vi "Acquire.vi"(8 "error in (no error)":errorcluster, 11 "DAQmxAI in":refnum<class "DAQmxAI.lvclass">) -> (0 "error out":errorcluster, 3 "DAQmxAI out":refnum<class "DAQmxAI.lvclass">)   [LabVIEW 2020, in "VolatusDAQ.lvlib" / "DAQmxAI.lvclass"]
uses:
  DAQmxAI.lvclass
  DAQmxAI.lvclass/DAQmxAI.ctl
  <vilib>/DAQmx/read.llb/DAQmx Read (Analog 1D Wfm NChan NSamp).vi
  <vilib>/DAQmx/miscellaneous.llb/DAQmx Fill In Error Info.vi
  VolatusData/VolatusData.lvlib
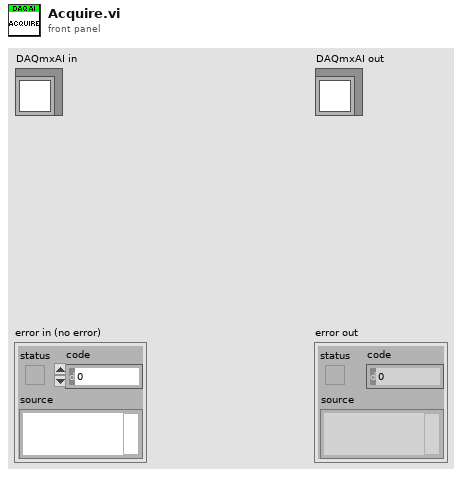
[diagram p1: front panel]
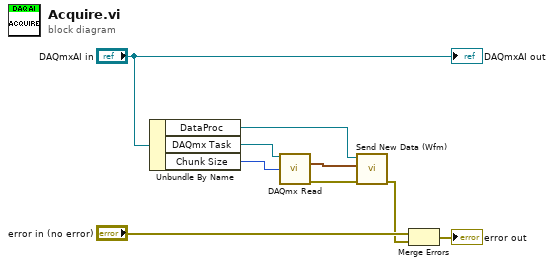
[diagram p0: block diagram]
diagram:
  n1 = Unbundle By Name("DAQmxAI in") -> ("DataProc"=w6:refnum<class "MessageQ.lvclass">, "DAQmx Task"=w8:refnum<k21>, "Chunk Size"=w7:i32)
  n2 = call-poly <vilib>:"DAQmx Read.vi"("task/channels in"=w8, "number of samples per channel"=w7) -> ("data"=w5:waveform(dbl)[], "error out"=w4:errorcluster)  [unwired: 11 in, 1 out]
  n3 = call "Send New Data (Wfm).vi"("error in (no error)"=w4, "Channels"=w5, "MessageQ"=w6) -> ("error out"=w1:errorcluster)  [unwired: 8 in]
  n4 = Merge Errors("error in (no error)", w1) -> (→"error out":errorcluster)
  "DAQmxAI out" <- "DAQmxAI in"
